vi "Read Nickname.vi"(8 "error in (no error)":errorcluster, 11 "Pele in":refnum<class "Pele.lvclass">) -> (0 "error out":errorcluster, 2 "Nickname":string, 3 "Pele out":refnum<class "Pele.lvclass">)   [LabVIEW 2019, in "Pele.lvclass"]
uses:
  Pele.lvclass
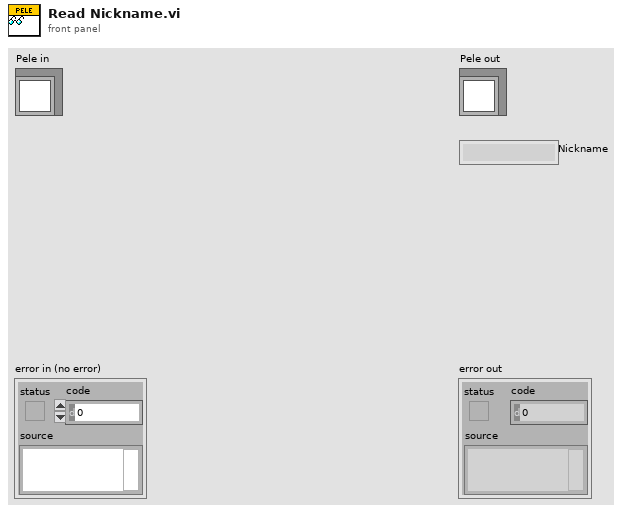
[diagram p1: front panel]
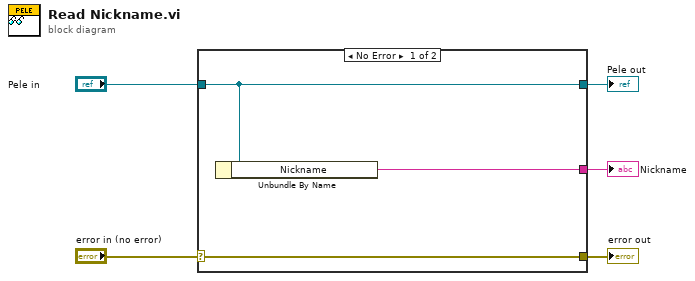
[diagram p0: block diagram]
diagram:
  n1 = case shown="No Error" "error in (no error)" {
    selector: "error in (no error)" -> [w8 w9]
    tunnel: [w8 w9] -> w4
    tunnel: [w7 w10] -> w2
    tunnel: "Pele in" -> [w7 w10]
    tunnel: [w6 _] -> w1
    frame No Error {
      n2 = Unbundle By Name(w7) -> ("Nickname"=w6:string)
    }
    frame Error {
    }
  }
  "error out" <- w4
  "Pele out" <- w2
  "Nickname" <- w1
